vi "law of cosines.vi"(9 "target to exit dist":dbl, 10 "center to target dist":dbl, 11 "center to exit dist":dbl) -> (3 "angle":dbl)   [LabVIEW 2019]
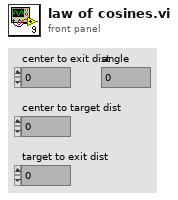
[diagram p1: front panel]
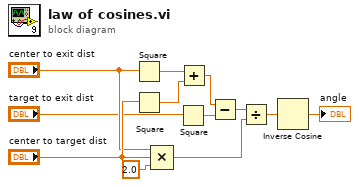
[diagram p0: block diagram]
diagram:
  n1 = Square(x="center to exit dist") -> (x^2=w2:dbl)
  n2 = Square(x="center to target dist") -> (x^2=w7:dbl)
  n3 = Compound Arithmetic op=MULTIPLY("center to exit dist", "center to target dist", 2.0 ("value")) -> (w9:dbl)
  n4 = Square(x="target to exit dist") -> (x^2=w4:dbl)
  n5 = Add(x=w2, y=w7) -> (x+y=w3:dbl)
  n6 = Subtract(x=w3, y=w4) -> (x-y=w8:dbl)
  n7 = Divide(x=w8, y=w9) -> (x/y=w10:dbl)
  n8 = Inverse Cosine(1:w10) -> (0:→"angle":dbl)
